vi "Generate Random Quaternion.vi"() -> (3 "random quaternion":T1)   [LabVIEW 2017, in "NI_Kinematics.lvlib"]
doc: "Returns a quaternion whose elements are between -1 and 1."
uses:
  <vilib>/robotics/Kinematics/NI_Kinematics.lvlib
  <vilib>/robotics/Kinematics/Quaternion.ctl
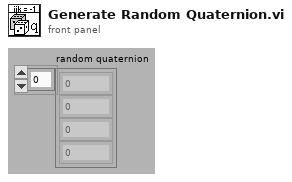
[diagram p1: front panel]
types:
  T1 = typedef "NI_Kinematics.lvlib/Quaternion.ctl" = dbl[]
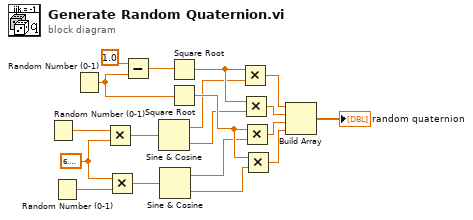
[diagram p0: block diagram]
diagram:
  w14 = 6.283185307179586
  n1 = Random Number (0-1)() -> (number: 0 to 1=w16:dbl)
  n2 = Random Number (0-1)() -> (number: 0 to 1=w15:dbl)
  n3 = Random Number (0-1)() -> (number: 0 to 1=w17:dbl)
  n4 = Multiply(x=w16, y=w14) -> (x*y=w13:dbl)
  n5 = Multiply(x=w14, y=w15) -> (x*y=w12:dbl)
  n6 = Subtract(x=1.0, y=w17) -> (x-y=w18:dbl)
  n7 = Sine & Cosine(0:w13) -> (1:w4:dbl, 2:w3:dbl)
  n8 = Sine & Cosine(0:w12) -> (1:w2:dbl, 2:w1:dbl)
  n9 = Square Root(x=w18) -> (sqrt(x)=w6:dbl)
  n10 = Square Root(x=w17) -> (sqrt(x)=w5:dbl)
  n11 = Multiply(x=w6, y=w4) -> (x*y=w9:dbl)
  n12 = Multiply(x=w6, y=w3) -> (x*y=w8:dbl)
  n13 = Multiply(x=w5, y=w2) -> (x*y=w7:dbl)
  n14 = Multiply(x=w5, y=w1) -> (x*y=w10:dbl)
  n15 = Build Array(w9, w8, w7, w10) -> (→"random quaternion":dbl[])
